vi "Inidces.vi"() -> ()   [LabVIEW 2019]
doc: "The myRIO Project template acquires acceleration data from the onboard accelerometer and displays the changes of acceleration values in a waveform chart."
uses:
  <vilib>/myRIO/Instrument Drivers/Onboard IO/DIO/typedefs/DIO Reference.ctl
  <vilib>/myRIO/Common/Instrument Driver Framework/Utilities/typedefs/myRIO Generic Hardware Reference.ctl
  <vilib>/myRIO/Common/Instrument Driver Framework/Utilities/typedefs/Hardware Version Enum.ctl
  <vilib>/myRIO/Common/Instrument Driver Framework/Utilities/typedefs/myRIO v1.0 Reference.ctl
  <vilib>/myRIO/Common/Instrument Driver Framework/Utilities/typedefs/Generic FPGA Reference.ctl
  <vilib>/myRIO/Common/Instrument Driver Framework/myRIO v1.0/DIO/typedefs/DIO Channels List.ctl
  <vilib>/myRIO/Common/Instrument Driver Framework/myRIO v1.0/DIO/typedefs/DIO Channels Enum.ctl
  <vilib>/userDefined/High Color/nirio_resource_hc.ctl
  <vilib>/myRIO/Instrument Drivers/Onboard IO/AI/typedefs/AI Reference.ctl
  <vilib>/myRIO/Common/Instrument Driver Framework/myRIO v1.0/AI/typedefs/AI Channels List.ctl
  <vilib>/myRIO/Common/Instrument Driver Framework/myRIO v1.0/AI/typedefs/AI Channels Enum.ctl
  <vilib>/myRIO/Common/Instrument Driver Framework/Utilities/typedefs/Analog Scaling Constants List.ctl
  <vilib>/myRIO/Common/Instrument Driver Framework/Utilities/typedefs/Analog Scaling Constants.ctl
  <vilib>/myRIO/Common/Instrument Driver Framework/Utilities/vis/Is FPGA Ref Available.vi
  <vilib>/myRIO/Common/Instrument Driver Framework/myRIO v1.0/DIO/vis/myRIO v1.1 Open DIO.vi
  <vilib>/myRIO/Instrument Drivers/Onboard IO/DIO/vis/Write.vi
  <vilib>/myRIO/Instrument Drivers/Onboard IO/DIO/vis/Read.vi
  <vilib>/myRIO/Common/Instrument Driver Framework/myRIO v1.0/AI/vis/myRIO v1.1 Open AI.vi
  <vilib>/myRIO/Instrument Drivers/Onboard IO/AI/vis/Read.vi
  <vilib>/myRIO/Common/Instrument Driver Framework/Utilities/vis/Validate Channels.vi
  <vilib>/myRIO/Common/Instrument Driver Framework/myRIO v1.0/DIO/vis/myRIO v1.0 Reserve DIO.vi
  <vilib>/myRIO/Common/Instrument Driver Framework/myRIO v1.0/AI/vis/myRIO v1.0 Reserve AI.vi
  <vilib>/myRIO/Common/Instrument Driver Framework/myRIO v1.0/UART/vis/myRIO v1.0 Close UART.vi
  <vilib>/myRIO/Common/Instrument Driver Framework/myRIO v1.0/Resource Manager/vis/myRIO v1.0 Reserve Channel List.vi
  <vilib>/myRIO/Common/Instrument Driver Framework/myRIO v1.0/DIO/vis/myRIO v1.0 Build MUX Configuration DIO.vi
  <vilib>/myRIO/Common/Instrument Driver Framework/myRIO v1.0/AI/vis/myRIO v1.0 Build MUX Configuration AI.vi
  <vilib>/myRIO/Common/Instrument Driver Framework/myRIO v1.0/Resource Manager/vis/myRIO v1.0 Reserve Channel.vi
  <vilib>/myRIO/Common/Instrument Driver Framework/myRIO v1.0/Resource Manager/vis/myRIO v1.0 Unreserve Channel.vi
  <vilib>/myRIO/Common/Instrument Driver Framework/myRIO v1.0/Resource Manager/vis/myRIO v1.0 Create Configuration List.vi
  <vilib>/myRIO/Common/Instrument Driver Framework/myRIO v1.0/Resource Manager/vis/myRIO v1.0 Build Mutex Name.vi
  <vilib>/Utility/VariantDataType/GetNumericInfo.vi
  <vilib>/Utility/error.llb/Error Cluster From Error Code.vi
  <vilib>/myRIO/Common/Instrument Driver Framework/myRIO v1.0/myRIO v1.1 Open.vi
  <vilib>/myRIO/Common/Instrument Driver Framework/Utilities/vis/IO Manager.vi
  <vilib>/myRIO/Common/Instrument Driver Framework/Utilities/vis/Configuration Manager.vi
  <vilib>/myRIO/Common/Instrument Driver Framework/myRIO v1.0/Resource Manager/vis/myRIO v1.0 Configure IO.vi
  <vilib>/myRIO/Common/Instrument Driver Framework/myRIO v1.0/myRIO v1.0 Close.vi
  <vilib>/myRIO/Common/Instrument Driver Framework/myRIO v1.0/DIO/vis/myRIO v1.0 Write DIO.vi
  <vilib>/myRIO/Common/Instrument Driver Framework/myRIO v1.0/DIO/vis/myRIO v1.0 Read DIO.vi
  <vilib>/myRIO/Common/Instrument Driver Framework/myRIO v1.0/AI/vis/myRIO v1.0 Get Scaling Constants AI.vi
  <vilib>/myRIO/Common/Instrument Driver Framework/myRIO v1.0/AI/vis/myRIO v1.0 Read AI.vi
  <vilib>/myRIO/Common/Instrument Driver Framework/Utilities/vis/FPGA Ref Manager.vi
  <vilib>/myRIO/Common/Instrument Driver Framework/myRIO v1.0/myRIO v1.0 Reset FPGA.vi
  <vilib>/myRIO/Common/Instrument Driver Framework/myRIO v1.0/IRQ/vis/myRIO v1.0 IRQ Info FGV.vi
  <vilib>/myRIO/Common/Instrument Driver Framework/myRIO v1.0/IRQ/vis/myRIO v1.0 Timer IRQ Info FGV.vi
  <vilib>/myRIO/Common/Instrument Driver Framework/myRIO v1.0/IRQ/vis/myRIO v1.0 ISR Agent.vi
  <vilib>/myRIO/Instrument Drivers/Utilities/vis/Reset Index.vi
  <vilib>/myRIO/Common/Instrument Driver Framework/myRIO v1.0/Resource Manager/vis/myRIO v1.0 Block Write Resource Manager.vi
  <vilib>/myRIO/Express VI/Onboard IO/DO/DO Express VI.xnode
  <vilib>/myRIO/Instrument Drivers/Onboard IO/DIO/vis/myRIO DIO Open.xnode
  <vilib>/myRIO/Express VI/Onboard IO/DI/DI Express VI.xnode
  <vilib>/myRIO/Express VI/Onboard IO/AI/AI Express VI.xnode
  <vilib>/myRIO/Instrument Drivers/Onboard IO/AI/vis/myRIO AI Open.xnode
  <vilib>/myRIO/Instrument Drivers/Onboard IO/DIO/DIO.lvlib
  <vilib>/myRIO/Instrument Drivers/Onboard IO/AI/AI.lvlib
  <vilib>/myRIO/Instrument Drivers/Utilities/Utilities.lvlib
panel:
  in  "Go":bool
  in  "Single/Continuous":bool
  out "INPOS":bool
  in  "Home":bool
  in  "OFF/ON":bool
  in  "L/R":bool
  out "Index":i8=-1
  in  "Displacement (cm)":u8(slide)=2 step=2 scale=0.0..10.0
  in  "Acceleration (m/s^2)":u8(slide)=1 min=1 max=5 step=1 scale=1.0..5.0
  out "Position (cm)":dbl(graph)
  out "error out":errorcluster
  in  "Stop":bool
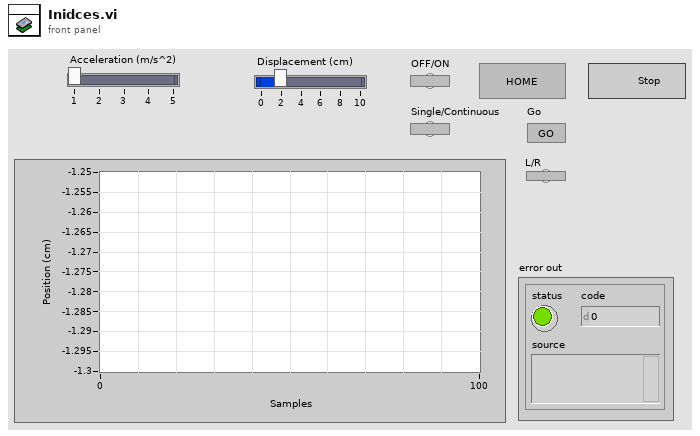
[diagram p1: front panel]
types:
  T1 = typedef "DIO.lvlib/DIO Reference.ctl" = cluster{"myRIO Reference":T2, "DIO Channels List":T6}
  T2 = typedef "myRIO Generic Hardware Reference.ctl" = cluster{"myRIO Model":T3, "myRIO Hardware Reference":T4}
  T3 = typedef "Hardware Version Enum.ctl" = enum16{"Unknown", "myRIO-1900", "myRIO-1950", "roboRIO", "NI ELVIS RIO CM", "ELVIS III"}
  T4 = typedef "myRIO v1.0 Reference.ctl" = cluster{"Generic FPGA Reference":T5, "Allow multiple opens":bool}
  T5 = typedef "Generic FPGA Reference.ctl" = refnum<k20>
  T6 = typedef "DIO Channels List.ctl" = T7[]
  T7 = typedef "DIO Channels Enum.ctl" = enum16{"Not Connected", "C/DIO0", "C/DIO1", "C/DIO2", "C/DIO3", "C/DIO4", "C/DIO5", "C/DIO6", "C/DIO7", "A/DIO0", "A/DIO1", "A/DIO2", "A/DIO3", "A/DIO4", "A/DIO5", "A/DIO6", "A/DIO7", "A/DIO8", "A/DIO9", "A/DIO10", "A/DIO11", "A/DIO12", "A/DIO13", "A/DIO14", "A/DIO15", "A/DIO16", "A/DIO17", "A/DIO18", "A/DIO19", "B/DIO0", "B/DIO1", "B/DIO2", "B/DIO3", "B/DIO4", "B/DIO5", "B/DIO6", "B/DIO7", "B/DIO8", "B/DIO9", "B/DIO10", "B/DIO11", "B/DIO12", "B/DIO13", "B/DIO14", "B/DIO15", "B/DIO16", "B/DIO17", "B/DIO18", "B/DIO19", "LED0", "LED1", "LED2", "LED3", "Button0", "DIO/DIO0", "DIO/DIO1", "DIO/DIO2", "DIO/DIO3", "DIO/DIO4", "DIO/DIO5", "DIO/DIO6", "DIO/DIO7", "DIO/DIO8", "DIO/DIO9", "SPI/CS0", "SPI/CS1", "SPI/CS2", "SPI/CS3", "LED RADIO (Green)", "LED RADIO (Red)", "LED COMM (Green)", "LED COMM (Red)", "LED MODE (Green)", "LED MODE (Red)"}
  T8 = typedef "nirio_resource_hc.ctl" = tag
  T9 = typedef "AI.lvlib/AI Reference.ctl" = cluster{"myRIO Reference":T2, "AI Channels List":T10, "AI Scaling Constants List":T12}
  T10 = typedef "AI Channels List.ctl" = T11[]
  T11 = typedef "AI Channels Enum.ctl" = enum16{"Not Connected", "AudioIn/Left", "AudioIn/Right", "C/AI0", "C/AI1", "A/AI0", "A/AI1", "A/AI2", "A/AI3", "A/AI4", "A/AI5", "A/AI6", "A/AI7", "B/AI0", "B/AI1", "B/AI2", "B/AI3", "B/AI4", "B/AI5", "B/AI6", "B/AI7", "AI/AI0", "AI/AI1", "AI/AI2", "AI/AI3", "A/AI0 (DIFF)", "A/AI1 (DIFF)", "A/AI2 (DIFF)", "A/AI3 (DIFF)", "B/AI0 (DIFF)", "B/AI1 (DIFF)", "B/AI2 (DIFF)", "B/AI3 (DIFF)"}
  T12 = typedef "Analog Scaling Constants List.ctl" = T13[]
  T13 = typedef "Analog Scaling Constants.ctl" = cluster{"LSB Weight (Volts)":dbl, "Offset (Volts)":dbl, "Signed?":bool}
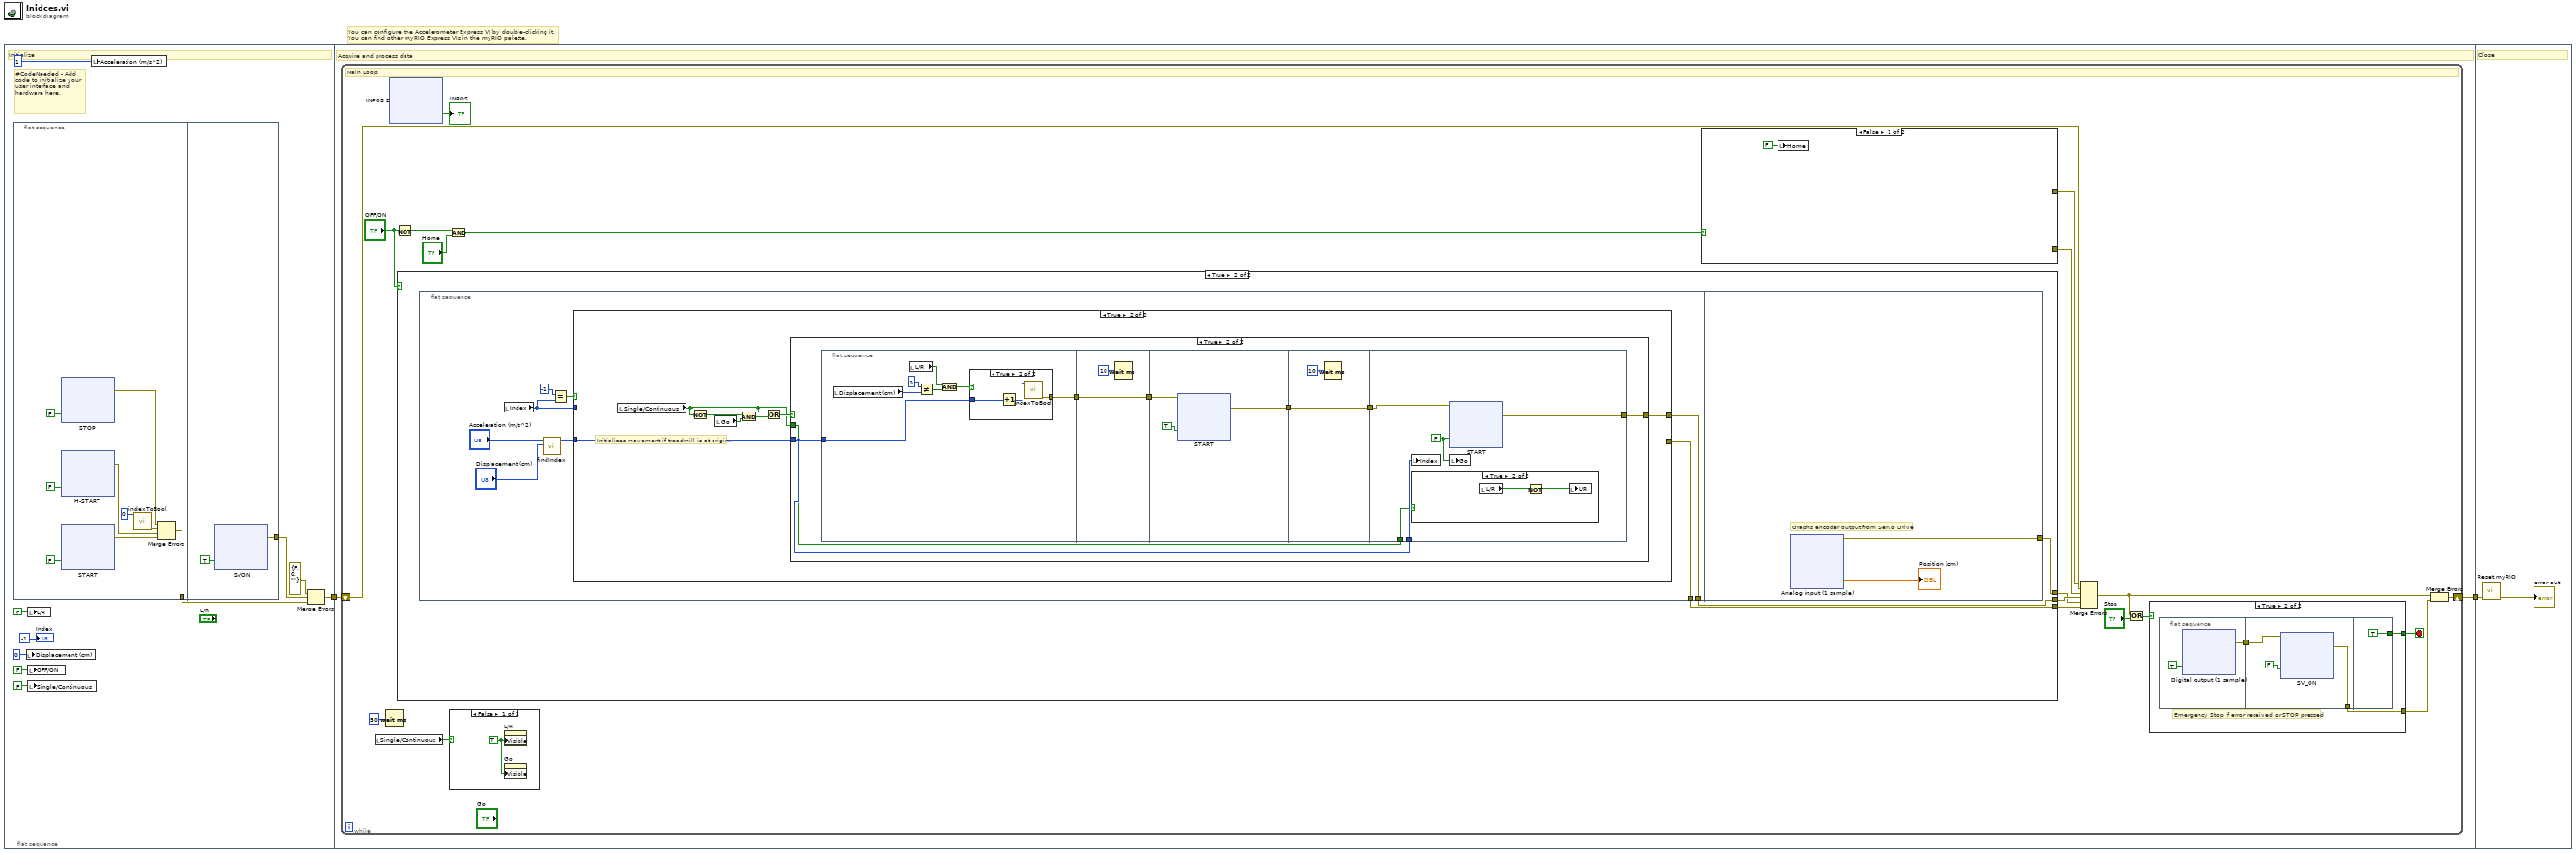
[diagram p0: block diagram]
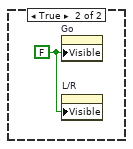
[diagram p2: hidden frame]
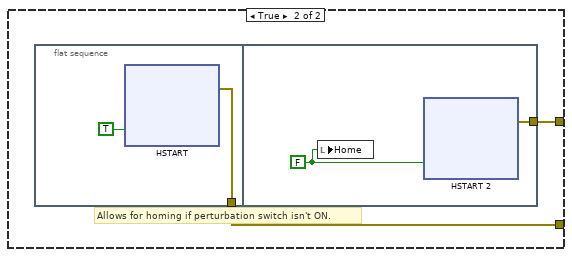
[diagram p4: hidden frame]
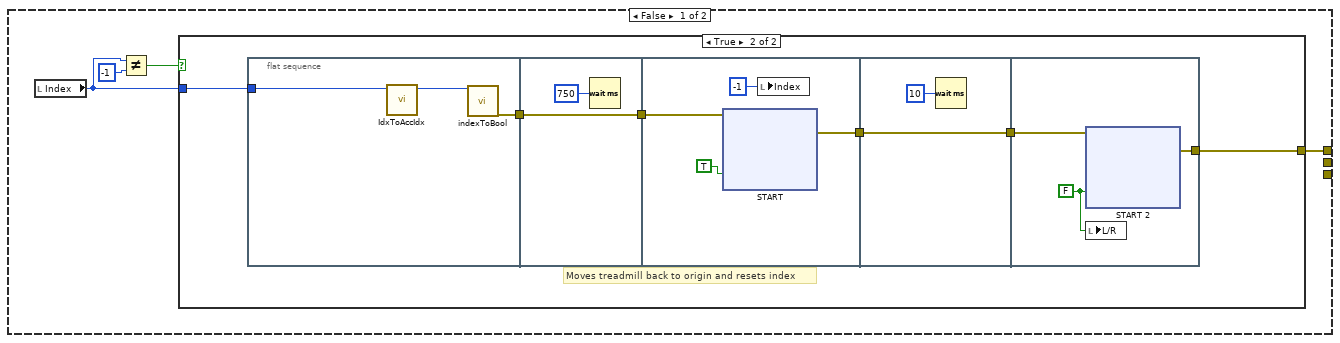
[diagram p5: hidden frame]
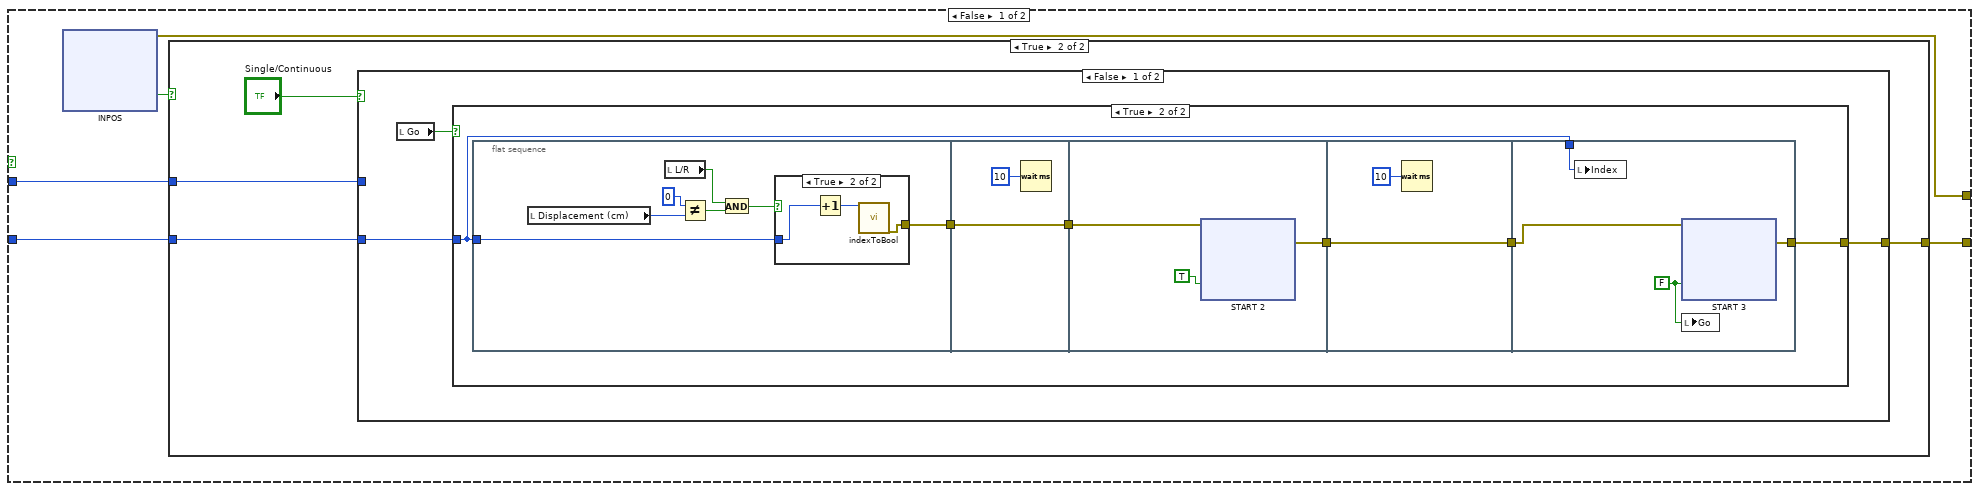
[diagram p7: hidden frame]
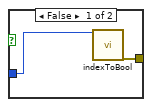
[diagram p10: hidden frame]
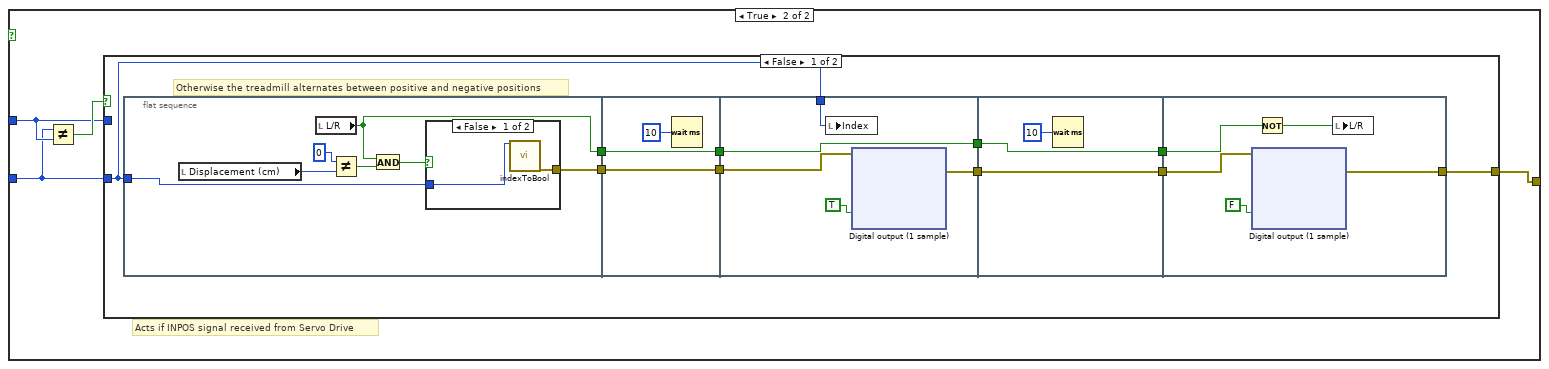
[diagram p11: hidden frame]
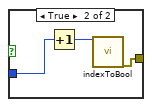
[diagram p12: hidden frame]
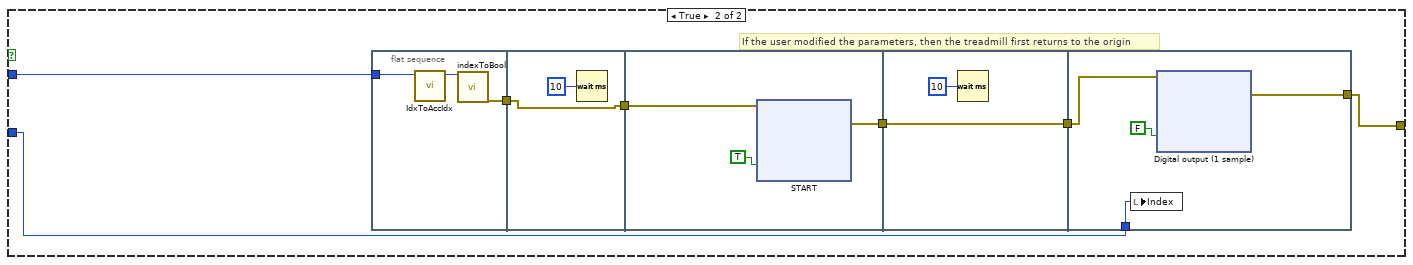
[diagram p13: hidden frame]
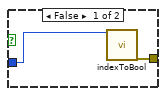
[diagram p15: hidden frame]
diagram:
  # "You can configure the Accelerometer Express VI by double-clicking it.\nYou can find other myRIO Express VIs in the myRIO palette."
  n1 = flat-sequence {
    tunnel: [w5] -> w2
    tunnel: w2 -> [w165]
    tunnel: [w164] -> w1
    tunnel: w1 -> [w981]
    frame #0 {
      # "#CodeNeeded - Add code to initialize your user interface and hardware here."
      # "Initialize"
      n2 = flat-sequence {
        tunnel: [w17] -> w7
        tunnel: [w128] -> w6
        frame #0 {
          n3 = xnode "STOP"("A/DIO0 (Pin 11)"=FALSE) -> ("error out"=w16:errorcluster)  [unwired: 1 in]
          n4 = xnode "H-START"("C/DIO3 (DIO3)"=FALSE) -> ("error out"=w19:errorcluster)  [unwired: 1 in]
          n5 = xnode "START"("C/DIO2 (DIO2)"=FALSE) -> ("error out"=w18:errorcluster)  [unwired: 1 in]
          n6 = call "indexToBool.vi"("Index"=0) -> ("error out"=w20:errorcluster)  [unwired: 18 in]
          n7 = Merge Errors(w16, w20, w19, w18) -> (w17:errorcluster)
        }
        frame #1 {
          n8 = xnode "SVON"("C/DIO1 (DIO1)"=TRUE) -> ("error out"=w128:errorcluster)  [unwired: 1 in]
        }
      }
      n9 = local write "Displacement (cm)"(0) -> ()
      n10 = local write "L/R"(FALSE) -> ()
      n11 = local write "OFF/ON"(FALSE) -> ()
      n12 = local write "Single/Continuous"(FALSE) -> ()
      n13 = local write "Acceleration (m/s^2)"(1) -> ()
      n14 = Merge Errors(errorcluster {"status"=FALSE, "code"=0, "source"=""} ("error in (no error)"), w6, w7) -> (w5:errorcluster)
      "Index" <- -1
    }
    frame #1 {
      # "Acquire and process data"
      n15 = while {
        shift-right: [w170] -> w164
        shift-left: w165 -> [w179]
        stop <- w173 stop-if-true
        # "Main Loop"
        n16 = local read "Single/Continuous"() -> (w166:bool)
        n17 = Wait (ms)(milliseconds to wait=u32 50) -> ()  [unwired: 1 out]
        n18 = xnode "INPOS 2"() -> ("C/DIO0 (DIO0)"=→"INPOS":bool)  [unwired: 1 in, 1 out]
        n19 = Not(x="OFF/ON") -> (.not. x?=w181:bool)
        n20 = case shown="True" "OFF/ON" {
          tunnel: [_ w474] -> w177
          tunnel: [w378 w473] -> w175
          tunnel: [_ w472] -> w168
          frame False {
            n21 = local read "Index"() -> (w379:i8)
            n22 = Not Equal?(x=w379, y=-1) -> (x != y?=w380:bool)
            n23 = case shown="True" w380 {
              tunnel: w379 -> [_ w387]
              tunnel: [_ w386] -> w378
              frame False {
              }
              frame True {
                # "Moves treadmill back to origin and resets index"
                n24 = flat-sequence {
                  tunnel: w387 -> [w389]
                  tunnel: [w388] -> w383
                  tunnel: w383 -> [w392]
                  tunnel: [w392] -> w382
                  tunnel: w382 -> [w395]
                  tunnel: [w394] -> w385
                  tunnel: w385 -> [w433]
                  tunnel: [w433] -> w384
                  tunnel: [w436] -> w386
                  tunnel: w384 -> [w435]
                  frame #0 {
                    n25 = call "IdxToAccIdx.vi"("Idx"=w389) -> ("Acc. Idx"=w390:u8)  [unwired: 9 in]
                    n26 = call "indexToBool.vi"("Index"=w390) -> ("error out"=w388:errorcluster)  [unwired: 18 in]
                  }
                  frame #1 {
                    n27 = Wait (ms)(milliseconds to wait=750) -> ()  [unwired: 1 out]
                  }
                  frame #2 {
                    n28 = xnode "START"("C/DIO2 (DIO2)"=TRUE, "error in (no error)"=w395) -> ("error out"=w394:errorcluster)
                    n29 = local write "Index"(-1) -> ()
                  }
                  frame #3 {
                    n30 = Wait (ms)(milliseconds to wait=10) -> ()  [unwired: 1 out]
                  }
                  frame #4 {
                    w434 = FALSE
                    n31 = xnode "START 2"("C/DIO2 (DIO2)"=w434, "error in (no error)"=w435) -> ("error out"=w436:errorcluster)
                    n32 = local write "L/R"(w434) -> ()
                  }
                }
              }
            }
          }
          frame True {
            n33 = flat-sequence {
              tunnel: [w477] -> w474
              tunnel: [w475] -> w472
              tunnel: [w942] -> w473
              frame #0 {
                n34 = local read "Index"() -> (w478:i8)
                n35 = call "findIndex.vi"("Disp."="Displacement (cm)", "Acc."="Acceleration (m/s^2)") -> ("Index"=w480:u8)  [unwired: 9 in]
                n36 = Equal?(x=-1, y=w478) -> (x = y?=w481:bool)
                n37 = case shown="True" w481 {
                  tunnel: w480 -> [w487 w838]
                  tunnel: w478 -> [w486 _]
                  tunnel: [w485 w837] -> w477
                  tunnel: [w484 _] -> w475
                  frame False {
                    n38 = xnode "INPOS"() -> ("C/DIO0 (DIO0)"=w483:bool, "error out"=w485:errorcluster)  [unwired: 1 in]
                    n39 = case shown="True" w483 {
                      tunnel: w487 -> [_ w525]
                      tunnel: w486 -> [_ w526]
                      tunnel: [_ w524] -> w484
                      frame False {
                      }
                      frame True {
                        n40 = case shown="False" "Single/Continuous" {
                          tunnel: w526 -> [_ w631]
                          tunnel: w525 -> [w529 w630]
                          tunnel: [w528 w629] -> w524
                          frame False {
                            n41 = local read "Go"() -> (w527:bool)
                            n42 = case shown="True" w527 {
                              tunnel: w529 -> [_ w531]
                              tunnel: [_ w530] -> w528
                              frame False {
                              }
                              frame True {
                                n43 = flat-sequence {
                                tunnel: w531 -> [w542]
                                tunnel: [w541] -> w535
                                tunnel: w535 -> [w549]
                                tunnel: [w549] -> w534
                                tunnel: w534 -> [w551]
                                tunnel: [w550] -> w533
                                tunnel: w533 -> [w589]
                                tunnel: [w589] -> w532
                                tunnel: w532 -> [w593]
                                tunnel: w531 -> [w592]
                                tunnel: [w591] -> w530
                                frame #0 {
                                n44 = local read "Displacement (cm)"() -> (w537:u8)
                                n45 = local read "L/R"() -> (w540:bool)
                                n46 = Not Equal?(x=0, y=w537) -> (x != y?=w538:bool)
                                n47 = And(x=w540, y=w538) -> (x .and. y?=w539:bool)
                                n48 = case shown="True" w539 {
                                tunnel: w542 -> [w543 w546]
                                tunnel: [w544 w547] -> w541
                                frame False {
                                n49 = call "indexToBool.vi"("Index"=w543) -> ("error out"=w544:errorcluster)  [unwired: 18 in]
                                }
                                frame True {
                                n50 = Increment(x=w546) -> (x+1=w545:u8)
                                n51 = call "indexToBool.vi"("Index"=w545) -> ("error out"=w547:errorcluster)  [unwired: 18 in]
                                }
                                }
                                }
                                frame #1 {
                                n52 = Wait (ms)(milliseconds to wait=10) -> ()  [unwired: 1 out]
                                }
                                frame #2 {
                                n53 = xnode "START 2"("C/DIO2 (DIO2)"=TRUE, "error in (no error)"=w551) -> ("error out"=w550:errorcluster)
                                }
                                frame #3 {
                                n54 = Wait (ms)(milliseconds to wait=10) -> ()  [unwired: 1 out]
                                }
                                frame #4 {
                                w590 = FALSE
                                n55 = local write "Index"(w592) -> ()
                                n56 = xnode "START 3"("C/DIO2 (DIO2)"=w590, "error in (no error)"=w593) -> ("error out"=w591:errorcluster)
                                n57 = local write "Go"(w590) -> ()
                                }
                                }
                              }
                            }
                          }
                          frame True {
                            # "Acts if INPOS signal received from Servo Drive"
                            n58 = Not Equal?(x=w630, y=w631) -> (x != y?=w632:bool)
                            n59 = case shown="False" w632 {
                              tunnel: w631 -> [_ w746]
                              tunnel: w630 -> [w642 w747]
                              tunnel: [w641 w745] -> w629
                              frame False {
                                # "Otherwise the treadmill alternates between positive and negative positions"
                                n60 = flat-sequence {
                                tunnel: [w646] -> w636
                                tunnel: w642 -> [w649]
                                tunnel: [w648] -> w634
                                tunnel: w636 -> [w657]
                                tunnel: [w657] -> w635
                                tunnel: w634 -> [w656]
                                tunnel: [w656] -> w633
                                tunnel: w642 -> [w662]
                                tunnel: [w661] -> w640
                                tunnel: w635 -> [w661]
                                tunnel: w633 -> [w659]
                                tunnel: [w658] -> w638
                                tunnel: w640 -> [w700]
                                tunnel: [w700] -> w639
                                tunnel: w638 -> [w699]
                                tunnel: [w699] -> w637
                                tunnel: w639 -> [w705]
                                tunnel: [w702] -> w641
                                tunnel: w637 -> [w701]
                                frame #0 {
                                n61 = local read "Displacement (cm)"() -> (w645:u8)
                                n62 = local read "L/R"() -> (w646:bool)
                                n63 = Not Equal?(x=0, y=w645) -> (x != y?=w643:bool)
                                n64 = And(x=w646, y=w643) -> (x .and. y?=w647:bool)
                                n65 = case shown="False" w647 {
                                tunnel: w649 -> [w650 w653]
                                tunnel: [w651 w654] -> w648
                                frame False {
                                n66 = call "indexToBool.vi"("Index"=w650) -> ("error out"=w651:errorcluster)  [unwired: 18 in]
                                }
                                frame True {
                                n67 = Increment(x=w653) -> (x+1=w652:u8)
                                n68 = call "indexToBool.vi"("Index"=w652) -> ("error out"=w654:errorcluster)  [unwired: 18 in]
                                }
                                }
                                }
                                frame #1 {
                                n69 = Wait (ms)(milliseconds to wait=10) -> ()  [unwired: 1 out]
                                }
                                frame #2 {
                                n70 = local write "Index"(w662) -> ()
                                n71 = xnode "Digital output (1 sample)"("C/DIO2 (DIO2)"=TRUE, "error in (no error)"=w659) -> ("error out"=w658:errorcluster)
                                }
                                frame #3 {
                                n72 = Wait (ms)(milliseconds to wait=10) -> ()  [unwired: 1 out]
                                }
                                frame #4 {
                                n73 = xnode "Digital output (1 sample)"("C/DIO2 (DIO2)"=FALSE, "error in (no error)"=w701) -> ("error out"=w702:errorcluster)
                                n74 = Not(x=w705) -> (.not. x?=w704:bool)
                                n75 = local write "L/R"(w704) -> ()
                                }
                                }
                              }
                              frame True {
                                # "If the user modified the parameters, then the treadmill first returns to the origin"
                                n76 = flat-sequence {
                                tunnel: w746 -> [w749]
                                tunnel: [w748] -> w742
                                tunnel: w742 -> [w752]
                                tunnel: [w752] -> w741
                                tunnel: w741 -> [w754]
                                tunnel: [w753] -> w743
                                tunnel: [w791] -> w744
                                tunnel: w743 -> [w791]
                                tunnel: w747 -> [w796]
                                tunnel: [w794] -> w745
                                tunnel: w744 -> [w793]
                                frame #0 {
                                n77 = call "IdxToAccIdx.vi"("Idx"=w749) -> ("Acc. Idx"=w750:u8)  [unwired: 9 in]
                                n78 = call "indexToBool.vi"("Index"=w750) -> ("error out"=w748:errorcluster)  [unwired: 18 in]
                                }
                                frame #1 {
                                n79 = Wait (ms)(milliseconds to wait=10) -> ()  [unwired: 1 out]
                                }
                                frame #2 {
                                n80 = xnode "START"("C/DIO2 (DIO2)"=TRUE, "error in (no error)"=w754) -> ("error out"=w753:errorcluster)
                                }
                                frame #3 {
                                n81 = Wait (ms)(milliseconds to wait=10) -> ()  [unwired: 1 out]
                                }
                                frame #4 {
                                n82 = local write "Index"(w796) -> ()
                                n83 = xnode "Digital output (1 sample)"("C/DIO2 (DIO2)"=FALSE, "error in (no error)"=w793) -> ("error out"=w794:errorcluster)
                                }
                                }
                              }
                            }
                          }
                        }
                      }
                    }
                  }
                  frame True {
                    # "Initializes movement if treadmill is at origin."
                    n84 = local read "Single/Continuous"() -> (w832:bool)
                    n85 = Not(x=w832) -> (.not. x?=w835:bool)
                    n86 = local read "Go"() -> (w834:bool)
                    n87 = And(x=w835, y=w834) -> (x .and. y?=w833:bool)
                    n88 = Or(x=w832, y=w833) -> (x .or. y?=w836:bool)
                    n89 = case shown="True" w836 {
                      tunnel: w838 -> [_ w841]
                      tunnel: [_ w840] -> w837
                      tunnel: w832 -> [_ w839]
                      frame False {
                      }
                      frame True {
                        n90 = flat-sequence {
                          tunnel: w841 -> [w851]
                          tunnel: [w852] -> w845
                          tunnel: w845 -> [w859]
                          tunnel: [w859] -> w844
                          tunnel: w844 -> [w861]
                          tunnel: [w860] -> w843
                          tunnel: w843 -> [w899]
                          tunnel: [w899] -> w842
                          tunnel: w841 -> [w904]
                          tunnel: [w903] -> w840
                          tunnel: w842 -> [w902]
                          tunnel: w839 -> [w900]
                          frame #0 {
                            n91 = local read "Displacement (cm)"() -> (w848:u8)
                            n92 = local read "L/R"() -> (w850:bool)
                            n93 = Not Equal?(x=0, y=w848) -> (x != y?=w847:bool)
                            n94 = And(x=w850, y=w847) -> (x .and. y?=w846:bool)
                            n95 = case shown="True" w846 {
                              tunnel: [w853 w857] -> w852
                              tunnel: w851 -> [w854 w855]
                              frame False {
                                n96 = call "indexToBool.vi"("Index"=w854) -> ("error out"=w853:errorcluster)  [unwired: 18 in]
                              }
                              frame True {
                                n97 = Increment(x=w855) -> (x+1=w856:u8)
                                n98 = call "indexToBool.vi"("Index"=w856) -> ("error out"=w857:errorcluster)  [unwired: 18 in]
                              }
                            }
                          }
                          frame #1 {
                            n99 = Wait (ms)(milliseconds to wait=10) -> ()  [unwired: 1 out]
                          }
                          frame #2 {
                            n100 = xnode "START"("C/DIO2 (DIO2)"=TRUE, "error in (no error)"=w861) -> ("error out"=w860:errorcluster)
                          }
                          frame #3 {
                            n101 = Wait (ms)(milliseconds to wait=10) -> ()  [unwired: 1 out]
                          }
                          frame #4 {
                            w901 = FALSE
                            n102 = local write "Index"(w904) -> ()
                            n103 = case shown="True" w900 {
                              frame False {
                              }
                              frame True {
                                n104 = local read "L/R"() -> (w905:bool)
                                n105 = Not(x=w905) -> (.not. x?=w906:bool)
                                n106 = local write "L/R"(w906) -> ()
                              }
                            }
                            n107 = xnode "START"("C/DIO2 (DIO2)"=w901, "error in (no error)"=w902) -> ("error out"=w903:errorcluster)
                            n108 = local write "Go"(w901) -> ()
                          }
                        }
                      }
                    }
                  }
                }
              }
              frame #1 {
                # "Graphs encoder output from Servo Drive"
                n109 = xnode "Analog input (1 sample)"() -> ("C/AI0 (AI0)"=→"Position (cm)":dbl, "error out"=w942:errorcluster)  [unwired: 1 in]
              }
            }
          }
        }
        n110 = case shown="False" w166 {
          frame False {
            w185 = TRUE
            n111 = property on="L/R" class="Bool (strict)"("Visible"=w185) -> ()  [unwired: 2 in, 2 out]
            n112 = property on="Go" class="Bool (strict)"("Visible"=w185) -> ()  [unwired: 2 in, 2 out]
          }
          frame True {
            w186 = FALSE
            n113 = property on="Go" class="Bool (strict)"("Visible"=w186) -> ()  [unwired: 2 in, 2 out]
            n114 = property on="L/R" class="Bool (strict)"("Visible"=w186) -> ()  [unwired: 2 in, 2 out]
          }
        }
        n115 = And(x=w181, y="Home") -> (x .and. y?=w182:bool)
        n116 = case shown="False" w182 {
          tunnel: [_ w303] -> w176
          tunnel: [_ w302] -> w167
          frame False {
            n117 = local write "Home"(FALSE) -> ()
          }
          frame True {
            # "Allows for homing if perturbation switch isn't ON."
            n118 = flat-sequence {
              tunnel: [w305] -> w303
              tunnel: [w342] -> w302
              frame #0 {
                n119 = xnode "HSTART"("C/DIO3 (DIO3)"=TRUE) -> ("error out"=w305:errorcluster)  [unwired: 1 in]
              }
              frame #1 {
                w341 = FALSE
                n120 = local write "Home"(w341) -> ()
                n121 = xnode "HSTART 2"("C/DIO3 (DIO3)"=w341) -> ("error out"=w342:errorcluster)  [unwired: 1 in]
              }
            }
          }
        }
        n122 = Merge Errors(w167, w179, w176, w177, w175, w168) -> (w172:errorcluster)
        n123 = Or(x=w172, y="Stop") -> (x .or. y?=w174:bool)
        n124 = case shown="True" w174 {
          tunnel: [_ w223] -> w173
          tunnel: [_ w224] -> w171
          frame False {
          }
          frame True {
            # "Emergency Stop if error received or STOP pressed"
            n125 = flat-sequence {
              tunnel: [w225] -> w222
              tunnel: [w264] -> w224
              tunnel: w222 -> [w262]
              tunnel: [TRUE] -> w223
              frame #0 {
                n126 = xnode "Digital output (1 sample)"("A/DIO0 (Pin 11)"=TRUE) -> ("error out"=w225:errorcluster)  [unwired: 1 in]
              }
              frame #1 {
                n127 = xnode "SV_ON"("C/DIO1 (DIO1)"=FALSE, "error in (no error)"=w262) -> ("error out"=w264:errorcluster)
              }
              frame #2 {
              }
            }
          }
        }
        n128 = Merge Errors(w172, w171) -> (w170:errorcluster)
      }
    }
    frame #2 {
      # "Close"
      n129 = call <vilib>:"Reset myRIO.vi"("error in (no error)"=w981) -> ("error out"=→"error out":errorcluster)  [unwired: 10 in]
    }
  }
